vi "Cascade MEMS Only Header Gen0 Ver1.1.vi"(8 "Error In":errorcluster, 11 "Select Design?":bool=TRUE) -> (0 "Error Out":errorcluster, 3 "Name Calculated Header":string[](array[string]))   [LabVIEW 2017]
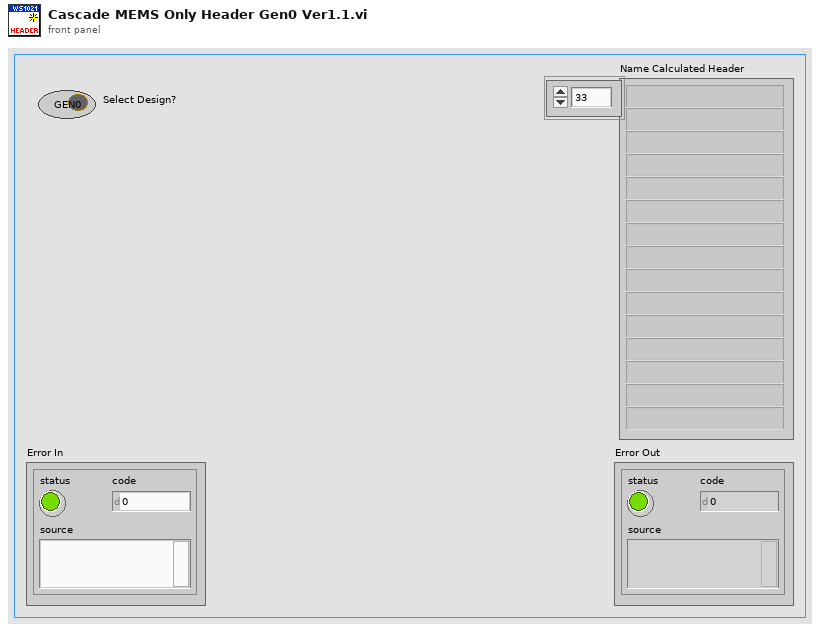
[diagram p1: front panel]
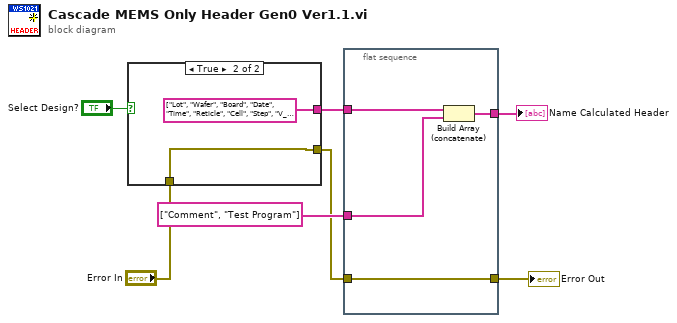
[diagram p0: block diagram]
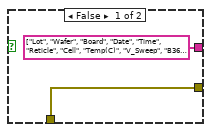
[diagram p2: hidden frame]
diagram:
  n1 = case shown="True" "Select Design?" {
    tunnel: [string[] ["Lot", "Wafer", "Board", "Date", "Time", "Reticle", "Cell", "Temp(C)", "V_Sweep", "B36_Up(fF)", "Delta B36 Up(fF)", "B36 DN(fF)", "Delta B36 DN(fF)", "B25 Up(fF)", "Delta B25 Up(fF)", "B25 DN(fF)", "Delta B25 DN(fF)", "12 Beams Up (fF)", "Delta 12 Beams Up(fF)", "12 Beams DN(fF)", "Delta 12 Beams DN(fF)", "%Delta B36 Up", "%Delta B36 DN", "%Delta B25 Up", "%Delta B25 DN", "%Delta 12 Beams Up", "%Delta 12 Beams DN"] string[] ["Lot", "Wafer", "Board", "Date", "Time", "Reticle", "Cell", "Step", "V_Sweep", "C1 Max(fF)", "Delta C1(fF)", "C3 Max(fF)", "Delta C3(fF)", "C4 Max(fF)", "Delta C4(fF)", "C2 Max(fF)", "Delta C2(fF)", "C5 Max(fF)", "Delta C5(fF)", "C6 Max(fF)", "Delta C6(fF)", "%Delta C1", "%Delta C3", "%Delta C4", "%Delta C2", "%Delta C5", "%Delta C6"]] -> w6
    tunnel: "Error In" -> [w9 w10]
    tunnel: [w9 w10] -> w1
    frame False {
    }
    frame True {
    }
  }
  n2 = flat-sequence {
    tunnel: w1 -> [w15]
    tunnel: [w15] -> w7
    tunnel: w6 -> [w14]
    tunnel: [w13] -> w5
    tunnel: string[] ["Comment", "Test Program"] -> [w12]
    frame #0 {
      n3 = Build Array (concatenate)(w14, w12) -> (w13:string[])
    }
  }
  "Name Calculated Header" <- w5
  "Error Out" <- w7
